vi "Config DS402 Drives.vi"(8 "error in (no error)":errorcluster, 10 "IOV Ref In":refnum<k21>, 11 "VS Ref In":T1=18446744073709551615 format="%.0x") -> (0 "error out":errorcluster, 2 "IOV Ref Out":refnum<k21>, 3 "VS Ref Out":T1=18446744073709551615 format="%.0x")   [LabVIEW 2016, in "Scan Engine Custom Device.lvlib"]
uses:
  Scan Engine Custom Device.lvlib
  <vilib>/NI Veristand/Custom Device API/Custom Device Item Ref.ctl
  <vilib>/NI Veristand/Custom Device API/Custom Device API.lvlib
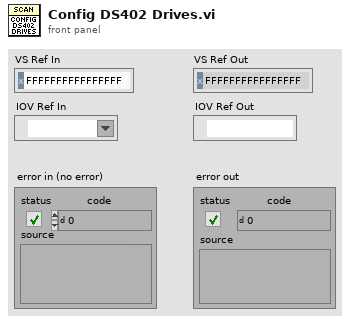
[diagram p1: front panel]
types:
  T1 = typedef "Custom Device API.lvlib/Custom Device Item Ref.ctl" = u64
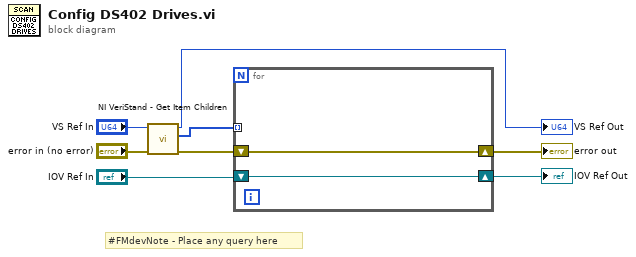
[diagram p0: block diagram]
diagram:
  # "#FMdevNote - Place any query here"
  n1 = call <vilib>:"NI VeriStand - Get Item Children.vi"("error in (no error)"="error in (no error)", "Item Ref in"="VS Ref In") -> ("error out"=w2:errorcluster, "Child Refs"=w1:T1[], "Item Ref out"=→"VS Ref Out":T1)  [unwired: 6 in, 1 out]
  n2 = for {
    shift-right: [w10] -> w4
    shift-left: w2 -> [w10]
    shift-right: [w9] -> w5
    shift-left: "IOV Ref In" -> [w9]
    tunnel: w1 -> [_] mode=indexing
  }
  "error out" <- w4
  "IOV Ref Out" <- w5
